vi "Teleop.vi"(10 "Match Info":T1={"Autonomous Elapsed Seconds"=0.0, "TeleOp Elapsed Seconds"=0.0, "Disabled Elapsed Seconds"=0.0, "Visited Autonomous"=FALSE, "Visited TeleOp"=FALSE, "Visited Disabled"=FALSE, "Autonomous Settings"={"Autonomous Style"=enum."Independent", "VI Refnum"=refnum}}, 11 "Call Context":T2) -> ()   [LabVIEW 2013]
doc: "This VI is called for each TeleOp packet received from the DS where the robot is not disabled. It is often used to read from the joysticks and update I/O or to update setpoints for timed control loops. It should complete and return within 20 milliseconds or it may miss DS packets."
uses:
  <vilib>/Rock Robotics/WPI/DriverStation/WPI_DriverStationDerivedRobotMode.ctl
  <vilib>/Rock Robotics/WPI/DriverStation/WPI_DriverStationMatch Info.ctl
  Robot Global Data.vi
  <vilib>/Rock Robotics/WPI/Joystick/WPI_JoystickGetSetRefNum.vi
panel:
  out "Numeric 1":dbl(slide) scale=0.0..100.0
  out "Boolean 2":bool
  out "Boolean 1":bool
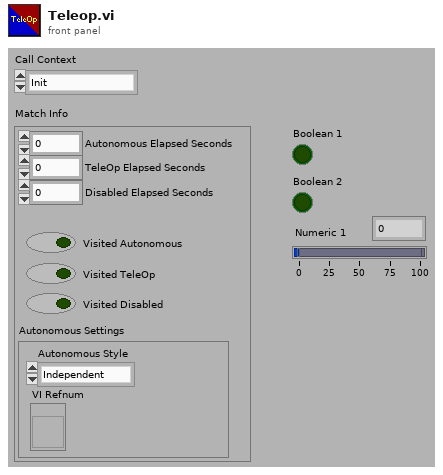
[diagram p1: front panel]
types:
  T1 = typedef "WPI_DriverStationMatch Info.ctl" = cluster{"Autonomous Elapsed Seconds":dbl, "TeleOp Elapsed Seconds":dbl, "Disabled Elapsed Seconds":dbl, "Visited Autonomous":bool, "Visited TeleOp":bool, "Visited Disabled":bool, "Autonomous Settings":cluster{"Autonomous Style":enum16{"Iterative", "Independent"}, "VI Refnum":refnum<vi>}}
  T2 = typedef "WPI_DriverStationDerivedRobotMode.ctl" = enum16{"Init", "Execute", "Stop"}
  T3 = typedef "User Commands typedef.ctl" = cluster{"Arm Command":T4, "Shooter Commands":T6, "Drive Commands":T7}
  T4 = typedef "Arm control typedef.ctl" = cluster{"Arm up/dwn":dbl, "Arm Capture":bool, "Arm Pass":bool, "Arm Positions":T5, "Arm Manual Override":bool}
  T5 = typedef "Arm Postions Enum Typedef.ctl" = enum16{"Arm Pick-up", "Arm Shoot", "Arm Truss"}
  T6 = typedef "Shooter Commands Typedef.ctl" = cluster{"Shooter Fire":bool, "Shooter Draw":bool}
  T7 = typedef "Drive Commands Typedef.ctl" = cluster{"Drive L/R":dbl, "Drive Fwd/Rev":dbl}
  T8 = typedef "WPI_JoystickDevRef.ctl" = cluster{"Device":T9}
  T9 = typedef "WPI_JoystickDeviceEnum.ctl" = enum16{"USB 1", "USB 2", "USB 3", "USB 4", "Kinect 1", "Kinect 2"}
  T10 = typedef "WPI_JoystickButtonState.ctl" = cluster{"Button 1":bool, "Button 2":bool, "Button 3":bool, "Button 4":bool, "Button 5":bool, "Button 6":bool, "Button 7":bool, "Button 8":bool, "Button 9":bool, "Button 10":bool, "Button 11":bool, "Button 12":bool}
  T11 = cluster{"axis 1 (x)":dbl, "axis 2 (y)":dbl, "axis 3 (throttle)":dbl, "axis 4":dbl, "axis 5":dbl, "axis 6":dbl}
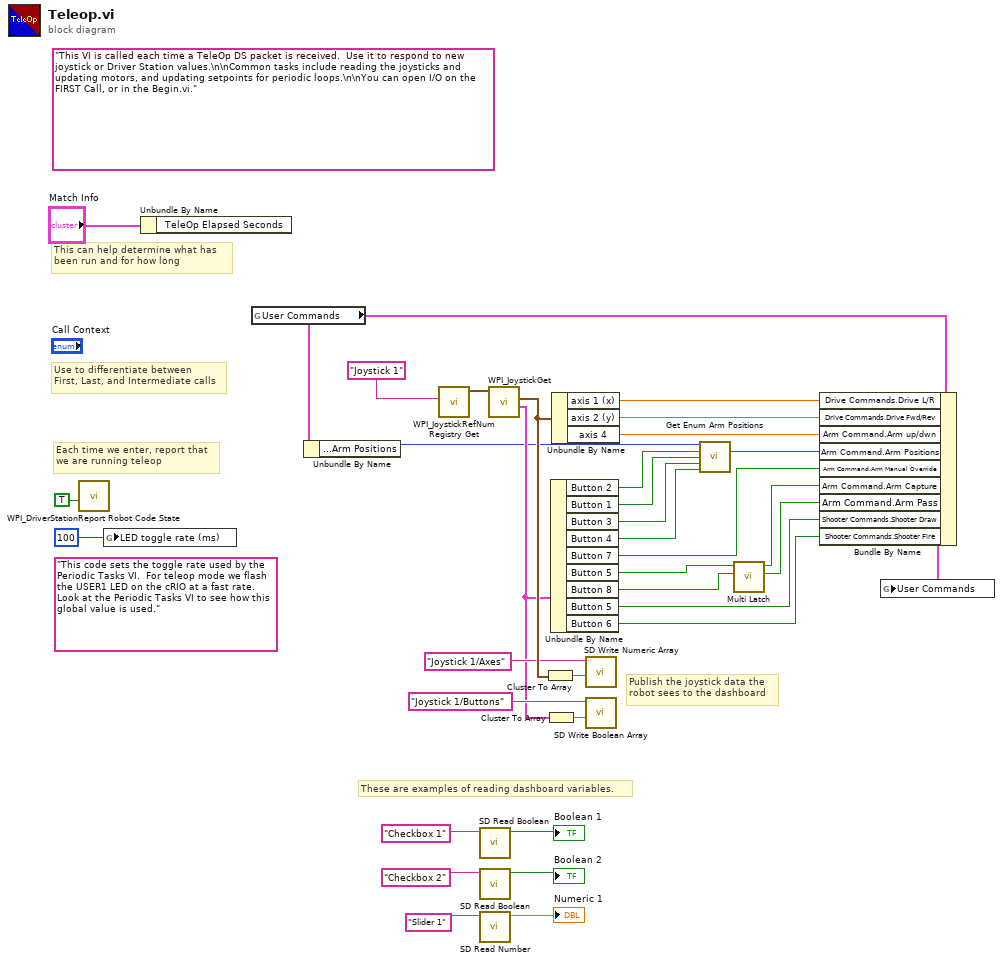
[diagram p0: block diagram]
diagram:
  (unwired) "This code sets the toggle rate used by the Periodic Tasks VI.  For teleop mode we flash the USER1 LED on the cRIO at a fast rate.  Look at the Periodic Tasks VI to see how this global value is used."
  (unwired) "This VI is called each time a TeleOp DS packet is received.  Use it to respond to new joystick or Driver Station values.\n\nCommon tasks include reading the joysticks and updating motors, and updating setpoints for periodic loops.\n\nYou can open I/O on the FIRST Call, or in the Begin.vi."
  # "These are examples of reading dashboard variables."
  # "Publish the joystick data the\nrobot sees to the dashboard"
  # "Each time we enter, report that\nwe are running teleop"
  # "Use to differentiate between\nFirst, Last, and Intermediate calls"
  # "This can help determine what has\nbeen run and for how long"
  n1 = call <vilib>:"WPI_DriverStationReport Robot Code State.vi"("TeleOp"=TRUE ("Autonomous")) -> ()  [unwired: 10 in, 1 out]
  n2 = global write "Robot Global Data.vi" "LED toggle rate (ms)"(u32 100 ("LED ms toggle rate")) -> ()
  n3 = Unbundle By Name("Match Info") -> ()  [unwired: 1 out]
  n4 = global read "Robot Global Data.vi" "User Commands"() -> (w13:T3)
  n5 = Unbundle By Name(w13) -> ("Arm Command.Arm Positions"=w12:T5)
  n6 = call <vilib>:"WPI_JoystickRefNum Registry Get.vi"("refnum name"="Joystick 1") -> ("JoystickDevRef"=w33:T8)  [unwired: 1 in, 9 out]
  n7 = call <vilib>:"SD Read Boolean.vi"("Name"="Checkbox 1" ("refnum name")) -> ("Boolean"=→"Boolean 1":bool)  [unwired: 8 in, 2 out]
  n8 = call <vilib>:"SD Read Boolean.vi"("Name"="Checkbox 2" ("refnum name")) -> ("Boolean"=→"Boolean 2":bool)  [unwired: 8 in, 2 out]
  n9 = call <vilib>:"SD Read Number.vi"("Name"="Slider 1" ("refnum name")) -> ("Numeric"=→"Numeric 1":dbl)  [unwired: 8 in, 2 out]
  n10 = call <vilib>:"WPI_JoystickGet.vi"("JoystickDevRef"=w33) -> ("Buttons"=w18:T10, "Axes"=w28:T11)  [unwired: 1 in, 4 out]
  n11 = Cluster To Array(cluster=w28) -> (array=w27:dbl[])
  n12 = Cluster To Array(cluster=w18) -> (array=w30:bool[])
  n13 = Unbundle By Name(w18) -> ("Button 2"=w9:bool, "Button 1"=w10:bool, "Button 3"=w11:bool, "Button 4"=w8:bool, "Button 7"=w17:bool, "Button 5"=w6:bool, "Button 8"=w5:bool, "Button 5"=w2:bool, "Button 6"=w1:bool)
  n14 = Unbundle By Name(w28) -> ("axis 1 (x)"=w16:dbl, "axis 2 (y)"=w15:dbl, "axis 4"=w14:dbl)
  n15 = call <vilib>:"SD Write Numeric Array.vi"("Numeric Array"=w27, "Name"="Joystick 1/Axes") -> ()  [unwired: 8 in, 2 out]
  n16 = call <vilib>:"SD Write Boolean Array.vi"("Boolean Array"=w30, "Name"="Joystick 1/Buttons") -> ()  [unwired: 8 in, 2 out]
  n17 = call "Get Enum Arm Positions.vi"("Previous Arm Position"=w12, "Pick-up Button"=w9, "Low Goal Button"=w10, "Shoot Button"=w11, "Trust Button"=w8) -> ("New Arm Position"=w7:T5)  [unwired: 10 in]
  n18 = call "Multi Latch.vi"("2"=w5, "1"=w6) -> ("2"=w3:bool, "1"=w4:bool)  [unwired: 6 in, 2 out]
  n19 = Bundle By Name(cluster=w13, "Drive Commands.Drive L/R"=w16, "Drive Commands.Drive Fwd/Rev"=w15, "Arm Command.Arm up/dwn"=w14, "Arm Command.Arm Positions"=w7, "Arm Command.Arm Manual Override"=w17, "Arm Command.Arm Capture"=w4, "Arm Command.Arm Pass"=w3, "Shooter Commands.Shooter Draw"=w2, "Shooter Commands.Shooter Fire"=w1) -> (w19:T3)
  n20 = global write "Robot Global Data.vi" "User Commands"(w19) -> ()
